vi "niDAQmx Set Channel Property.vi"   [LabVIEW 2021, in "Session Management niDAQmx.lvlib" / "Session Factory.lvclass"]
doc: "Property node to set information to NI-DAQmx channels."
uses:
  Session Factory.lvclass
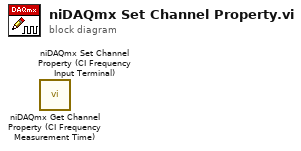
[diagram p0: block diagram]
diagram:
  n1 = call "niDAQmx Get Channel Property (CI Frequency Measurement Time).vi"() -> ()  [unwired: 13 in, 3 out]
  n2 = call "niDAQmx Set Channel Property (CI Frequency Input Terminal).vi"() -> ()  [unwired: 14 in, 2 out]
